vi "全局 1.vi"() -> ()   [LabVIEW 2011]
panel:
  in  "setting":T1
  out "9dots":dbl[][](array[numeric])
  out "ScaleArray":T2
  out "AdjustFactor":T3
  out "eyemovement":dbl[](array[numeric])
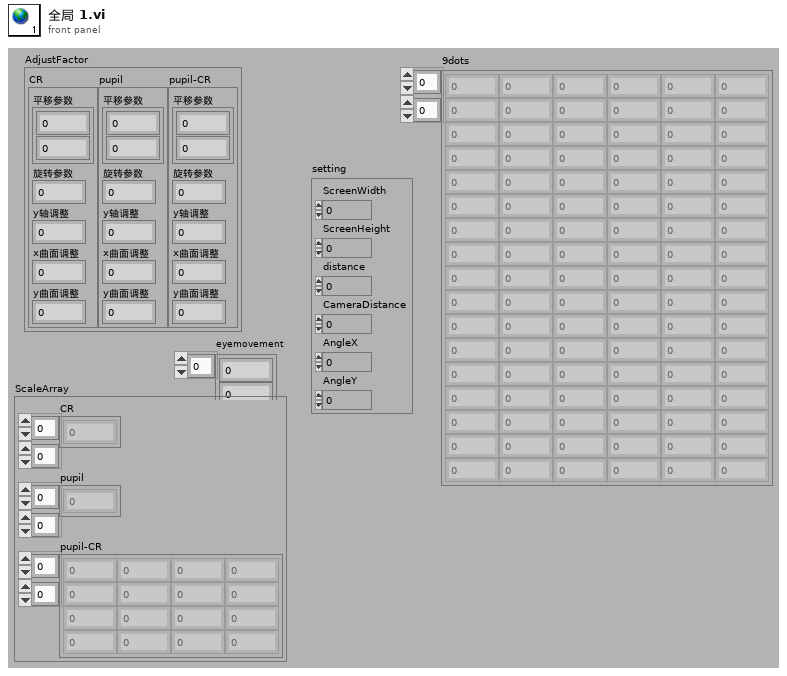
[diagram p1: front panel]
types:
  T1 = cluster{"ScreenWidth":i32, "ScreenHeight":i32, "distance":i32, "CameraDistance":i32, "AngleX":i32, "AngleY":i32}
  T2 = cluster{"CR":dbl[][], "pupil":dbl[][], "pupil-CR":dbl[][]}
  T3 = cluster{"CR":cluster{"平移参数":cluster{dbl, dbl}, "旋转参数":dbl, "y轴调整":dbl, "x曲面调整":dbl, "y曲面调整":dbl}, "pupil":cluster{"平移参数":cluster{dbl, dbl}, "旋转参数":dbl, "y轴调整":dbl, "x曲面调整":dbl, "y曲面调整":dbl}, "pupil-CR":cluster{"平移参数":cluster{dbl, dbl}, "旋转参数":dbl, "y轴调整":dbl, "x曲面调整":dbl, "y曲面调整":dbl}}
diagram:
